vi "inference_http.vi"() -> ()   [LabVIEW 2021]
uses:
  <vilib>/httpClient/POSTBuffer.vi
  <vilib>/httpClient/LabVIEWHTTPClient.lvlib
panel:
  out "concatenated string":string
  out "body":string
  out "headers":string
  out "data_path_string":string
  out "Application Directory":path
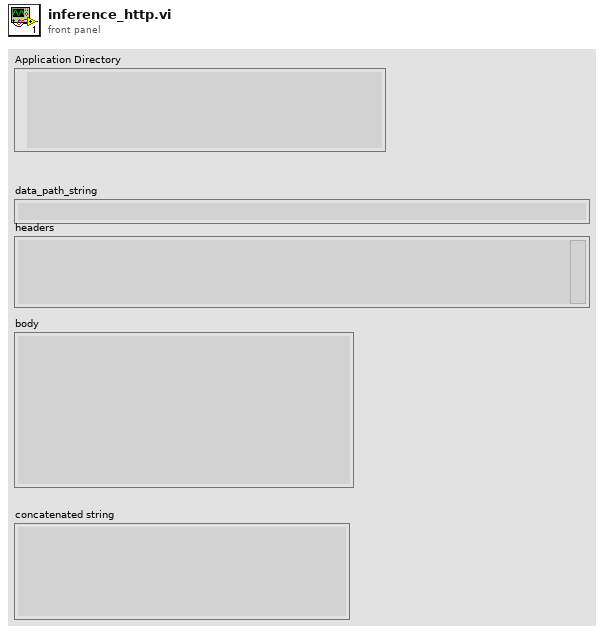
[diagram p1: front panel]
types:
  T1 = typedef "LabVIEWHTTPClient.lvlib/ClientHandle.ctl" = refnum<k1>
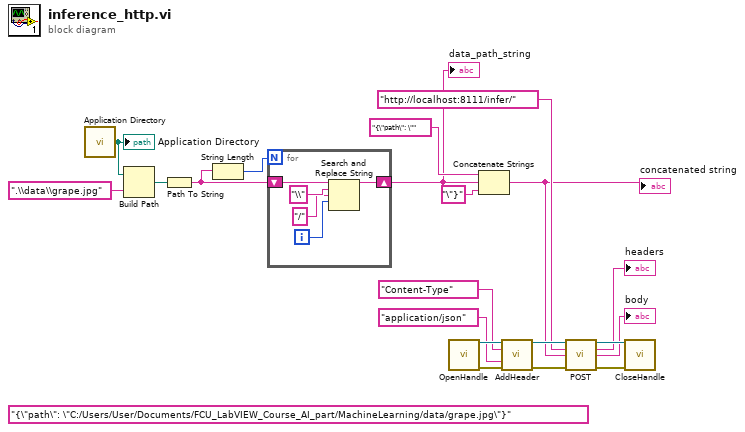
[diagram p0: block diagram]
diagram:
  (unwired) "{\"path\": \"C:/Users/User/Documents/FCU_LabVIEW_Course_AI_part/MachineLearning/data/grape.jpg\"}" ("buffer")
  n1 = call <vilib>:"Application Directory.vi"() -> ("Application Directory"=w18:path)
  "Application Directory" <- w18
  n2 = Build Path(base path=w18, name or relative path=".\\data\\grape.jpg") -> (appended path=w19:path)
  n3 = Path To String(path=w19) -> (string=w16:string)
  n4 = String Length(string=w16) -> (length=w17:i32)
  n5 = for {
    N: w17 -> [_]
    shift-right: [w21] -> w2
    shift-left: w16 -> [w24]
    i -> [w22]
    n6 = Search and Replace String(input string=w24, search string="\\", replace string="/" ("replace string (\"\")"), offset=w22) -> (result string=w21:string)  [unwired: 4 in, 3 out]
  }
  "data_path_string" <- w2
  n7 = call <vilib>:"OpenHandle.vi"() -> ("client handle out"=w11:T1, "error out"=w10:errorcluster)  [unwired: 14 in]
  n8 = Concatenate Strings("{\"path\": \"" ("string"), w2, "\"}" ("string")) -> (w1:string)
  "concatenated string" <- w1
  n9 = call <vilib>:"AddHeader.vi"("client handle"=w11, "header"="Content-Type", "value"="application/json", "error in (no error)"=w10) -> ("client handle out"=w9:T1, "error out"=w8:errorcluster)  [unwired: 10 in]
  n10 = call-poly <vilib>:"POST.vi"("client handle"=w9, "url"="http://localhost:8111/infer/", "buffer"=w1, "error in (no error)"=w8) -> ("client handle out"=w15:T1, "headers"=→"headers":string, "body"=→"body":string, "error out"=w14:errorcluster)  [unwired: 8 in]
  n11 = call <vilib>:"CloseHandle.vi"("client handle"=w15, "error in (no error)"=w14) -> ()  [unwired: 13 in, 1 out]
